vi "GEA2 Write ERD Multiple Messages.vi"(0 "GEA2 Reference In":refnum<k24>, 1 "# of Tries":u8=3 min=1 step=1, 2 "Read Timeout (ms)":u32=500, 5 "GEA Inputs":T1 {"Destination" format="%.0x"; "Source" format="%.0x"}, 7 "Write ERD List":T2[](array[typedef]) {"ERD Number" format="%.0x"}, 11 "Error In":errorcluster, 12 "#ERDs per message":i32=1 min=1 step=1, 13 "Verify ERD Response?":bool=TRUE) -> (4 "GEA2 Reference Out":refnum<k24>, 8 "Raw Data Out":string[](array[string]), 15 "Error Out":errorcluster)   [LabVIEW 2020, in "GEA2_Toolkit.lvlib"]
uses:
  library/GEA2_Toolkit.lvlib
  type defs/ERD Write Data In.ctl
  type defs/Data Type.ctl
  C:/TechnologyLab/NI-2010/Drivers/GEA3 Toolkit/GEA3 DLL Source/GeaCommunication.dll
  GEA3 DLL Source/GeaCommunication.dll
  type defs/Source_Destination.ctl
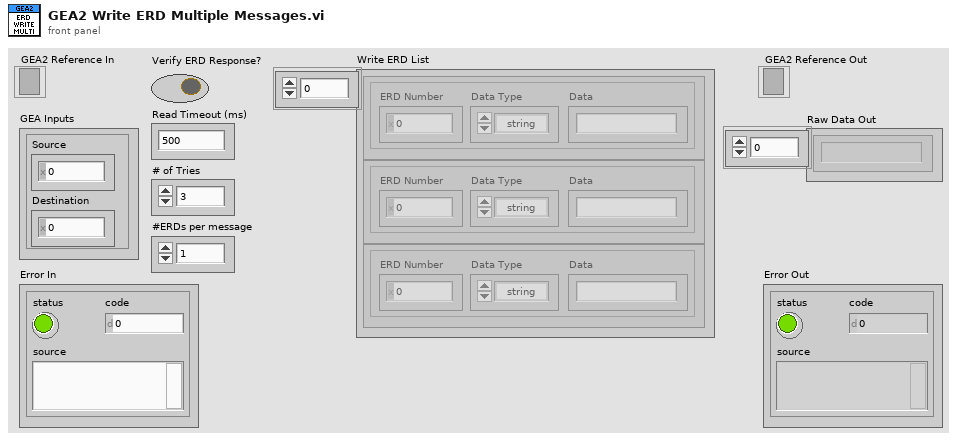
[diagram p1: front panel]
types:
  T1 = typedef "GEA2_Toolkit.lvlib/Source_Destination.ctl" = cluster{"Source":u8, "Destination":u8}
  T2 = typedef "GEA2_Toolkit.lvlib/ERD Write Data In.ctl" = cluster{"ERD Number":u16, "Data Type":T3, "Data":string}
  T3 = typedef "GEA2_Toolkit.lvlib/Data Type.ctl" = enum16{"string", "boolean", "uint8_t", "uint16_t", "uint32_t", "uint64_t", "int8_t", "int16_t", "int32_t", "int64_t"}
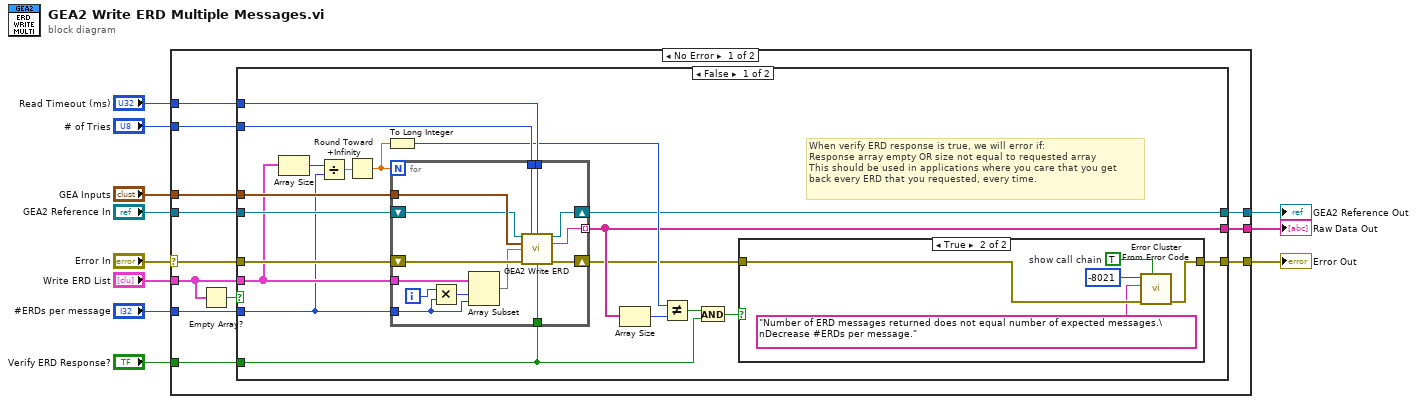
[diagram p0: block diagram]
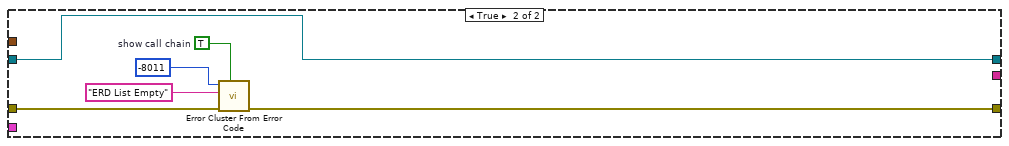
[diagram p3: hidden frame]
diagram:
  n1 = case shown="No Error" "Error In" {
    selector: "Error In" -> [w12 w70]
    tunnel: [w23 w69] -> w11
    tunnel: [w22 w70] -> w10
    tunnel: "Verify ERD Response?" -> [w21 _]
    tunnel: "GEA Inputs" -> [w20 _]
    tunnel: "Read Timeout (ms)" -> [w19 _]
    tunnel: "# of Tries" -> [w18 _]
    tunnel: "GEA2 Reference In" -> [w17 w69]
    tunnel: "#ERDs per message" -> [w16 _]
    tunnel: [w15 _] -> w3
    tunnel: "Write ERD List" -> [w13 _]
    frame No Error {
      n2 = Empty Array?(array=w13) -> (empty?=w14:bool)
      n3 = case shown="False" w14 {
        tunnel: [w27 w63] -> w23
        tunnel: w12 -> [w42 w65]
        tunnel: [w31 w64] -> w22
        tunnel: w21 -> [w26 _]
        tunnel: w20 -> [w41 _]
        tunnel: w19 -> [w40 _]
        tunnel: w18 -> [w39 _]
        tunnel: w17 -> [w38 w63]
        tunnel: w13 -> [w36 _]
        tunnel: w16 -> [w35 _]
        tunnel: [w29 _] -> w15
        frame False {
          # "When verify ERD response is true, we will error if:\nResponse array empty OR size not equal to requested array\nThis should be used in applications where you care that you get\nback every ERD that you requested, every time."
          n4 = Array Size(array=w36) -> (size(s)=w34:i32)
          n5 = Divide(x=w34, y=w35) -> (x/y=w37:dbl)
          n6 = Round Toward +Infinity(x=w37) -> (ceil(x): smallest int >= x=w33:dbl)
          n7 = To Long Integer(number=w33) -> (32bit integer=w30:i32)
          n8 = for {
            N: w33 -> [_]
            tunnel: w26 -> [w59]
            tunnel: w41 -> [w58]
            tunnel: [w57] -> w29 mode=indexing
            tunnel: w40 -> [w56]
            tunnel: w39 -> [w49]
            shift-right: [w62] -> w27
            shift-left: w38 -> [w50]
            shift-right: [w60] -> w28
            shift-left: w42 -> [w61]
            tunnel: w36 -> [w55]
            tunnel: w35 -> [w54]
            i -> [w53]
            n9 = Multiply(x=w53, y=w54) -> (x*y=w52:i32)
            n10 = Array Subset(array=w55, index=w52, length=w54) -> (w51:T2[])
            n11 = call "GEA2 Write ERD.vi"("GEA2 Reference In"=w50, "# of Tries"=w49, "Read Timeout (ms)"=w56, "GEA Inputs"=w58, "Write ERD List"=w51, "Error In"=w61, "Verify ERD Response?"=w59) -> ("GEA2 Reference Out"=w62:refnum<k24>, "Raw Data Out"=w57:string, "Error Out"=w60:errorcluster)  [unwired: 6 in]
          }
          n12 = Array Size(array=w29) -> (size(s)=w32:i32)
          n13 = Not Equal?(x=w30, y=w32) -> (x != y?=w24:bool)
          n14 = And(x=w24, y=w26) -> (x .and. y?=w25:bool)
          n15 = case shown="True" w25 {
            tunnel: w28 -> [w43 w46]
            tunnel: [w43 w45] -> w31
            frame False {
            }
            frame True {
              w48 = TRUE  # show call chain
              n16 = call <vilib>:"Error Cluster From Error Code.vi"("show call chain? (False)"=w48, "error in (no error)"=w46, "error message (\"\")"="Number of ERD messages returned does not equal number of expected messages.\nDecrease #ERDs per message." ("error message (\"\")"), "error code (0)"=-8021) -> ("error out"=w45:errorcluster)  [unwired: 5 in]
            }
          }
        }
        frame True {
          w66 = TRUE  # show call chain
          n17 = call <vilib>:"Error Cluster From Error Code.vi"("show call chain? (False)"=w66, "error in (no error)"=w65, "error message (\"\")"="ERD List Empty" ("error message (\"\")"), "error code (0)"=-8011) -> ("error out"=w64:errorcluster)  [unwired: 5 in]
        }
      }
    }
    frame Error {
    }
  }
  "GEA2 Reference Out" <- w11
  "Error Out" <- w10
  "Raw Data Out" <- w3
